vi "v1h_get_NC_vararray.vi"(3 "error in (no error)":errorcluster caption="错误输入（无错误）", 4 "NC_dimarray":cluster{"name":string, "size":u64}[](array[cluster]), 5 "refnum in":refnum<file>) -> (0 "error out":errorcluster, 1 "NC_vararray":T1(array[cluster]), 2 "refnum out":refnum<file>)   [LabVIEW 2016]
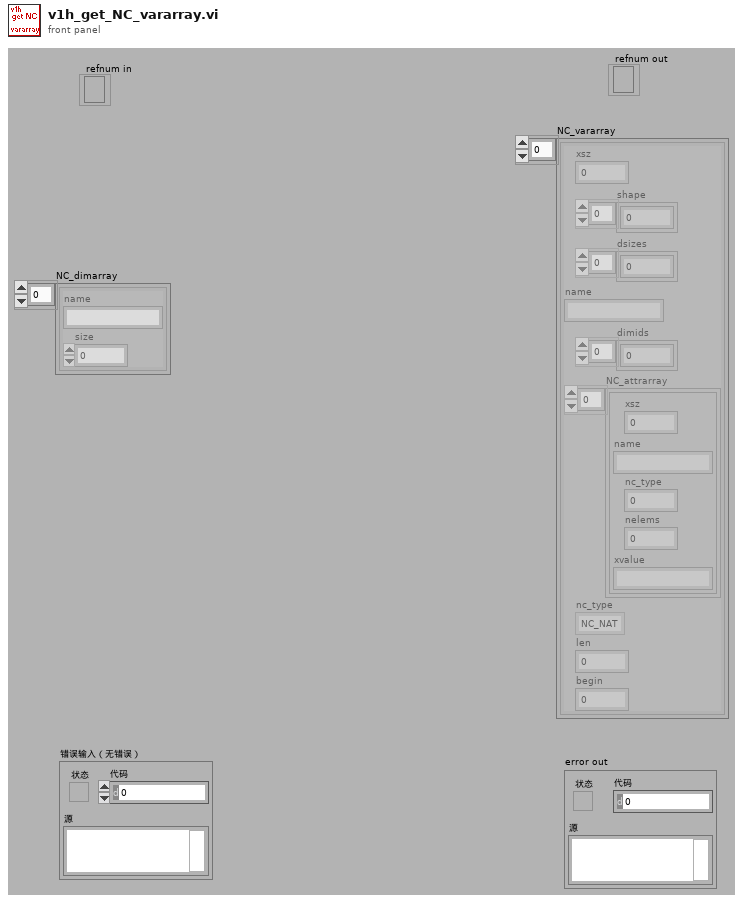
[diagram p1: front panel]
types:
  T1 = cluster{"xsz":u64, "shape":u64[], "dsizes":u64[], "name":string, "dimids":u64[], "NC_attrarray":cluster{"xsz":u64, "name":string, "nc_type":u16, "nelems":u64, "xvalue":string}[], "nc_type":enum16{"NC_NAT", "NC_BYTE", "NC_CHAR", "NC_SHORT", "NC_INT", "NC_FLOAT", "NC_DOUBLE"}, "len":u64, "begin":u64}[]
  T2 = cluster{"xsz":u64, "shape":u64[], "dsizes":u64[], "name":string, "dimids":u64[], "NC_attrarray":cluster{"xsz":u64, "name":string, "nc_type":u16, "nelems":u64, "xvalue":string}[], "nc_type":enum16{"NC_NAT", "NC_BYTE", "NC_CHAR", "NC_SHORT", "NC_INT", "NC_FLOAT", "NC_DOUBLE"}, "len":u64, "begin":u64}
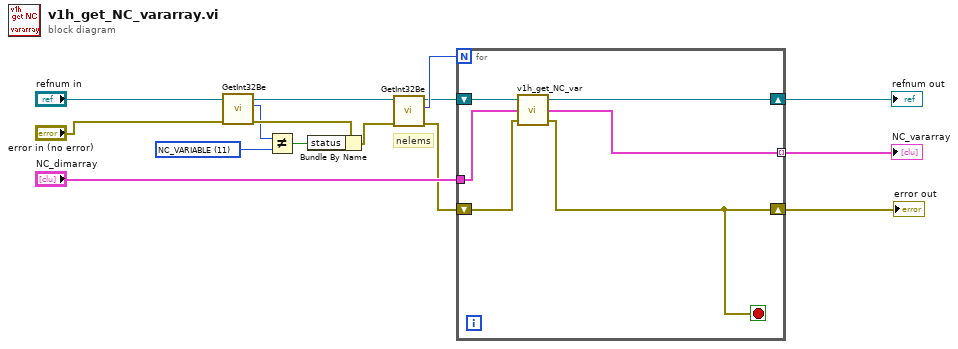
[diagram p0: block diagram]
diagram:
  w7 = u16 11 items=["NC_UNSPECIFIED"=0, "NC_BITFIELD"=7, "NC_STRING"=8, "NC_DIMENSION"=10, "NC_VARIABLE"=11, "NC_ATTRIBUTE"=12] ("NCtype")
  # "nelems"
  n1 = call "GetInt32Be.vi"("error in (no error)"="error in (no error)", "refnum in"="refnum in") -> ("error out"=w8:errorcluster, "int32"=w6:i32, "refnum out"=w10:refnum<file>)  [unwired: 3 out]
  n2 = Not Equal?(x=w6, y=w7) -> (x != y?=w9:bool)
  n3 = Bundle By Name(cluster=w8, "status"=w9) -> (w11:errorcluster)
  n4 = call "GetInt32Be.vi"("error in (no error)"=w11, "refnum in"=w10) -> ("error out"=w3:errorcluster, "int32"=w13:i32, "refnum out"=w12:refnum<file>)  [unwired: 3 out]
  n5 = for {
    N: w13 -> [_]
    shift-right: [w21] -> w5
    shift-left: w12 -> [w17]
    tunnel: "NC_dimarray" -> [w18]
    tunnel: [w20] -> w1 mode=indexing
    shift-right: [w16] -> w2
    shift-left: w3 -> [w19]
    stop <- w16 stop-if-true
    n6 = call "v1h_get_NC_var.vi"("error in (no error)"=w19, "NC_dimarray"=w18, "refnum in"=w17) -> ("error out"=w16:errorcluster, "NC_var"=w20:T2, "refnum out"=w21:refnum<file>)
  }
  "NC_vararray" <- w1
  "refnum out" <- w5
  "error out" <- w2
